vi "Voltage To Diode Create.vi"(8 "error in (no error)":errorcluster, 11 "Top in":refnum<class "Top.lvclass">) -> (0 "error out":errorcluster, 3 "Top out":refnum<class "Top.lvclass">)   [LabVIEW 2021, in "Top.lvlib" / "Top.lvclass"]
uses:
  Top.lvclass
  <vilib>/NathanCo/Analog Tasks/Utilities/Analog Configuration Parameters.ctl
  Top.lvclass/Top.ctl
  <vilib>/NathanCo/Analog Tasks/Analog Output/Analog Output/Analog Output.lvclass
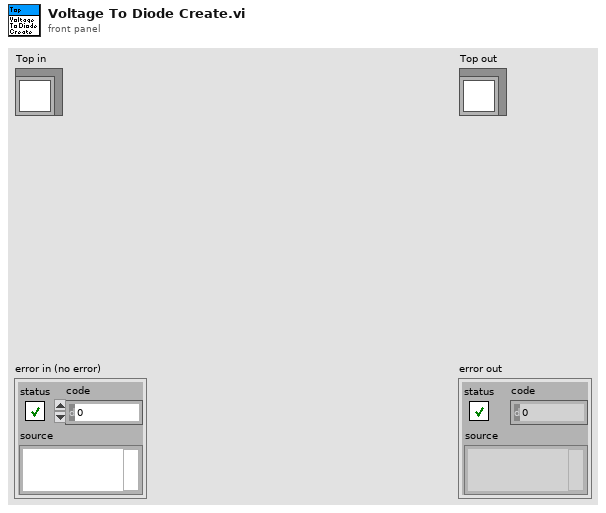
[diagram p1: front panel]
types:
  T1 = typedef "Analog Configuration Parameters.ctl" = cluster{"Terminal Configuration":i32, "Minimum Voltage":dbl, "Maximum Voltage":dbl, "Simulated?":bool, "Device":string, "Device Number":string, "Channel":string, "NI_ChannelName":string}
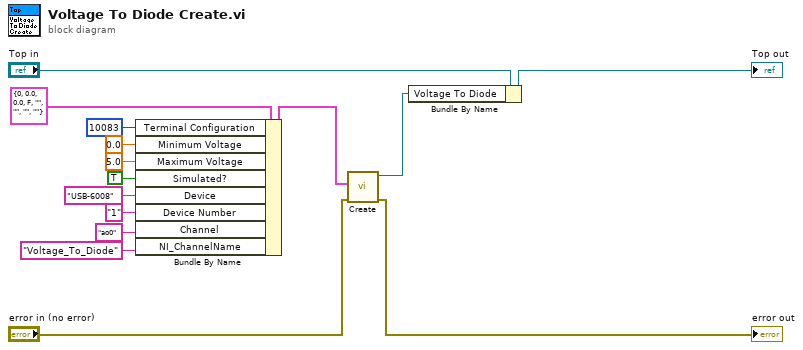
[diagram p0: block diagram]
diagram:
  n1 = Bundle By Name(cluster=T1 {"Terminal Configuration"=0, "Minimum Voltage"=0.0, "Maximum Voltage"=0.0, "Simulated?"=FALSE, "Device"="", "Device Number"="", "Channel"="", "NI_ChannelName"=""} ("Analog_Configuration_Parameters"), "Terminal Configuration"=10083, "Minimum Voltage"=0.0, "Maximum Voltage"=5.0, "Simulated?"=TRUE, "Device"="USB-6008", "Device Number"="1", "Channel"="ao0", "NI_ChannelName"="Voltage_To_Diode") -> (w9:T1)
  n2 = call <vilib>:"Create.vi"("error in (no error)"="error in (no error)", "Analog_Configuration_Parameters"=w9) -> ("error out"=→"error out":errorcluster, "Analog Output out"=w13:refnum<class "Analog Output.lvclass">)  [unwired: 8 in]
  n3 = Bundle By Name(cluster="Top in", "Voltage To Diode"=w13) -> (→"Top out":refnum<class "Top.lvclass">)
